vi "fill.vi"(7 "depth":i32[][](array[numeric]), 8 "index":i32, 9 "col":i32, 10 "row":i32, 11 "basins":i32[][](array[numeric])) -> (3 "basins out":i32[][](array[numeric]))   [LabVIEW 2017]
uses:
  eec96c2a-fc57-43e1-b73a-f5e48168438b.vi
  <vilib>/Utility/Debug Log/Display.vi
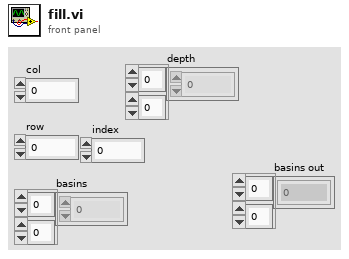
[diagram p1: front panel]
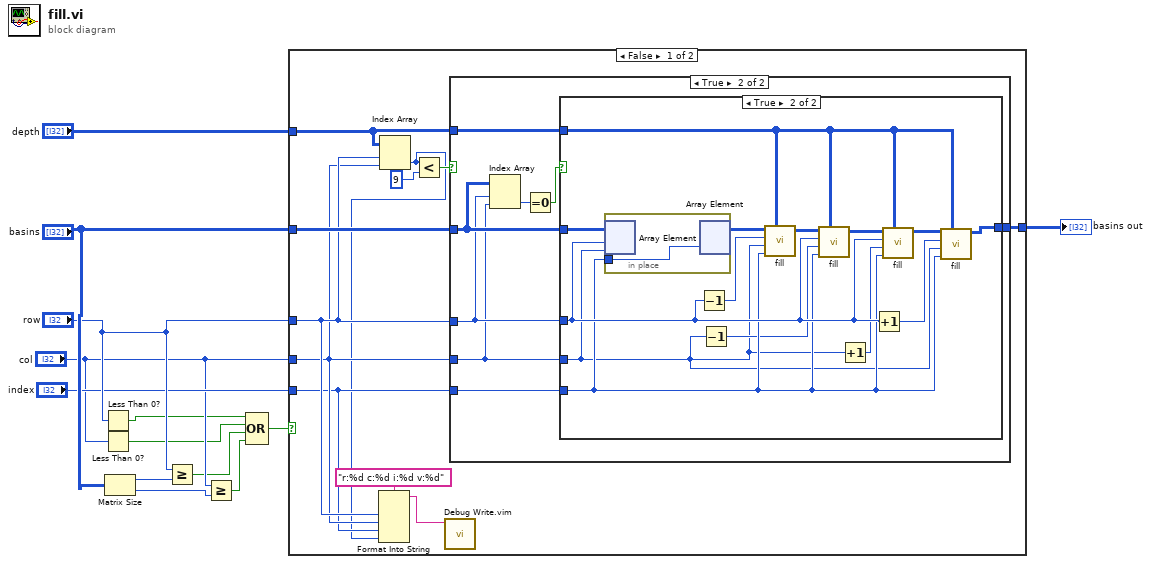
[diagram p0: block diagram]
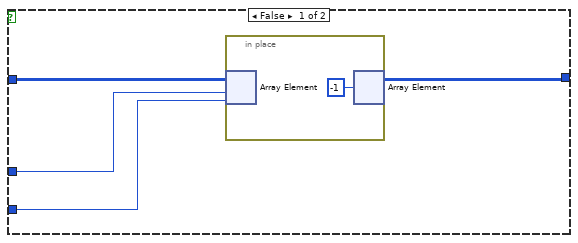
[diagram p2: hidden frame]
diagram:
  n1 = Less Than 0?(x="row") -> (x < 0?=w5:bool)
  n2 = Less Than 0?(x="col") -> (x < 0?=w4:bool)
  n3 = Matrix Size(0:"basins") -> (1:w9:i32, 2:w6:i32)
  n4 = Greater Or Equal?(x="row", y=w9) -> (x >= y?=w3:bool)
  n5 = Greater Or Equal?(x="col", y=w6) -> (x >= y?=w2:bool)
  n6 = Compound Arithmetic op=OR(w5, w4, w3, w2) -> (w1:bool)
  n7 = case shown="False" w1 {
    tunnel: [w24 w54] -> w13
    tunnel: "depth" -> [w23 _]
    tunnel: "basins" -> [w21 w54]
    tunnel: "row" -> [w19 _]
    tunnel: "index" -> [w17 _]
    tunnel: "col" -> [w18 _]
    frame False {
      n8 = Index Array(array=w23, index (row)=w19, index (col)=w18) -> (element=w14:i32)
      n9 = Format Into String(format string="r:%d c:%d i:%d v:%d", w19, w18, w17, w14) -> (resulting string=w16:string)  [unwired: 2 in, 1 out]
      n10 = Less?(x=w14, y=9) -> (x < y?=w15:bool)
      n11 = call "Debug Write.vim"("value"=w16) -> ()  [unwired: 10 in, 1 out]
      n12 = case shown="True" w15 {
        tunnel: [w27 w37] -> w24
        tunnel: w23 -> [_ w36]
        tunnel: w21 -> [w28 w35]
        tunnel: w19 -> [w26 w33]
        tunnel: w18 -> [w25 w30]
        tunnel: w17 -> [_ w32]
        frame False {
          n13 = in-place {
            n14 = in-place-array #1(w28, w26, w25) -> ()  [unwired: 1 out]
            n15 = in-place-array #1(-1 ("element")) -> (w27:i32[][])  [unwired: 2 out]
          }
        }
        frame True {
          n16 = Index Array(array=w35, index (row)=w33, index (col)=w30) -> (element=w34:i32)
          n17 = Equal To 0?(x=w34) -> (x = 0?=w31:bool)
          n18 = case shown="True" w31 {
            tunnel: [w38 w52] -> w37
            tunnel: w36 -> [_ w47]
            tunnel: w35 -> [w38 w46]
            tunnel: w33 -> [_ w44]
            tunnel: w32 -> [_ w43]
            tunnel: w30 -> [_ w39]
            frame False {
            }
            frame True {
              n19 = in-place {
                in-place-border: w43 -> [w53]
                n20 = in-place-array #2(w46, w44, w39) -> ()  [unwired: 1 out]
                n21 = in-place-array #2(w53) -> (w48:i32[][])  [unwired: 2 out]
              }
              n22 = Decrement(x=w44) -> (x-1=w42:i32)
              n23 = Decrement(x=w39) -> (x-1=w41:i32)
              n24 = call "fill.vi"("depth"=w47, "index"=w43, "col"=w39, "row"=w42, "basins"=w48) -> ("basins out"=w49:i32[][])  [unwired: 6 in]
              n25 = call "fill.vi"("depth"=w47, "index"=w43, "col"=w41, "row"=w44, "basins"=w49) -> ("basins out"=w50:i32[][])  [unwired: 6 in]
              n26 = Increment(x=w39) -> (x+1=w40:i32)
              n27 = Increment(x=w44) -> (x+1=w45:i32)
              n28 = call "fill.vi"("depth"=w47, "index"=w43, "col"=w40, "row"=w44, "basins"=w50) -> ("basins out"=w51:i32[][])  [unwired: 6 in]
              n29 = call "fill.vi"("depth"=w47, "index"=w43, "col"=w39, "row"=w45, "basins"=w51) -> ("basins out"=w52:i32[][])  [unwired: 6 in]
            }
          }
        }
      }
    }
    frame True {
    }
  }
  "basins out" <- w13
